vi "Run Alicat Configuration.vi"(8 "error in (no error)":errorcluster, 11 "Alicat Device in":refnum<class "Alicat Device.lvclass">) -> (0 "error out":errorcluster, 1 "value":dbl, 2 "Accessors:controller_":bool, 3 "Alicat Device out":refnum<class "Alicat Device.lvclass">)   [LabVIEW 2014, in "Alicat Lib.lvlib" / "Alicat Device.lvclass"]
uses:
  Alicat Device.lvclass
  reusable/Session APIs/Serial/Serial Session.lvclass
  Data/Alicat Data.lvclass
  Configurable Device/Configurable Device.lvclass/Configurable Device.ctl
  reusable/Data/Data.lvclass/Data.ctl
  Data/Alicat Data.lvclass/Alicat Data.ctl
  Alicat Device.lvclass/Alicat Device.ctl
  reusable/Session APIs/File Access/Config Data/Config Data.lvclass/Config Data.ctl
  Configurable Device/Accessors/Write label.vi
  Accessors/Read Session Handle.vi
  Configurable Device/Read controller_.vi
  Accessors/Write Session Handle.vi
  Configurable Device/Accessors/Write type.vi
  reusable/Data/Write Data ID.vi
  Data/Accessors/Write ID.vi
  Configurable Device/Read Handle.vi
  Configurable Device/Read Log Session.vi
  <vilib>/Utility/config.llb/Read Key (String).vi
  <vilib>/Utility/config.llb/Read Key (Double).vi
  reusable/Session APIs/File Access/Config Data/Config Data.lvclass
  <userlib>/_Session Fwk/Session - Root.lvclass
  <vilib>/ErrorRing/Error Ring.xnode
  <vilib>/Utility/config.llb/NI_LVConfig.lvlib
  Configurable Device/Configurable Device.lvclass
  reusable/Session APIs/Session Log/System Log.lvclass
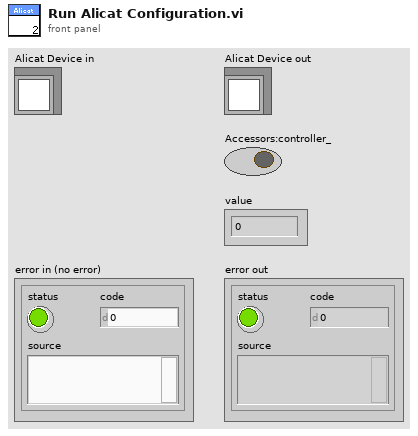
[diagram p1: front panel]
types:
  T1 = typedef "Serial Session.lvclass/Session Handle.ctl" = refnum<data-value>
  T2 = typedef "Config Data.lvclass/Config Session.ctl" = refnum<data-value>
  T3 = typedef "Session - Root.lvclass/Session Handle.ctl" = refnum<data-value>
  T4 = typedef "NI_LVConfig.lvlib/Config Data RefNum.ctl" = refnum<k1>
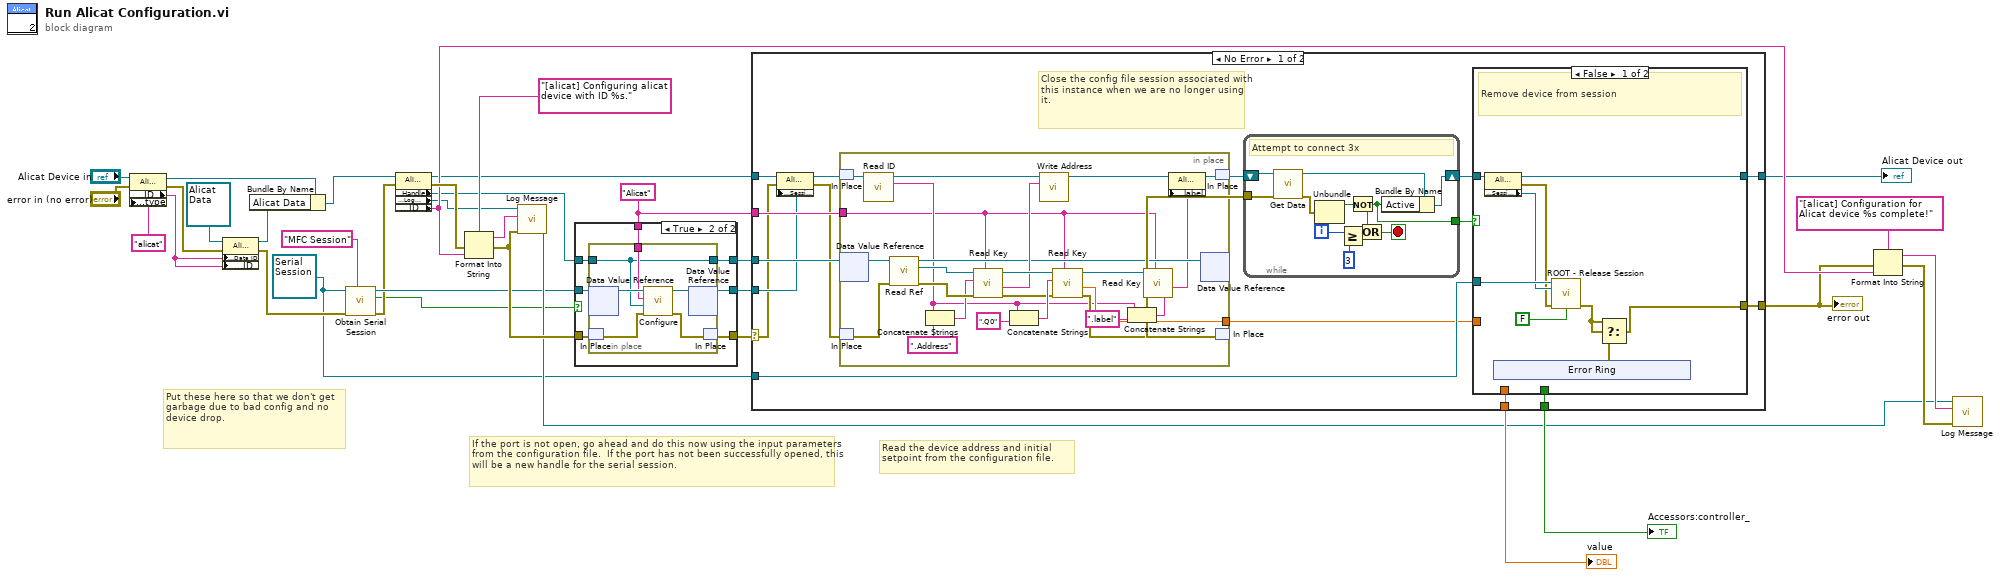
[diagram p0: block diagram]
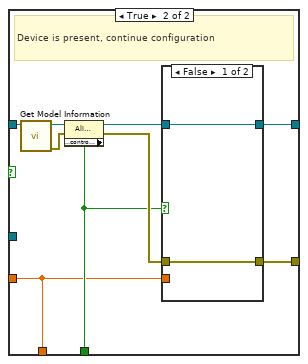
[diagram p2: hidden frame]
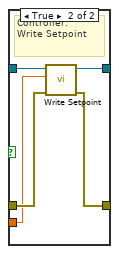
[diagram p3: hidden frame]
diagram:
  w8 = refnum<class "Serial Session.lvclass"> refnum ("Serial Session in")
  w6 = "Alicat" ("section")
  # "Put these here so that we don't get garbage due to bad config and no device drop."
  # "If the port is not open, go ahead and do this now using the input parameters from the configuration file.  If the port has not been successfully opened, this will be a new handle for the serial session."
  # "Read the device address and initial setpoint from the configuration file."
  n1 = property class="Alicat Device"(reference="Alicat Device in", error in="error in (no error)", "Accessors:type"="alicat" ("type")) -> (reference out=w24:refnum<class "Alicat Device.lvclass">, error out=w27:errorcluster, "Accessors:ID"=w23:string)
  n2 = property class="Alicat Data"(reference=refnum<class "Alicat Data.lvclass"> refnum ("Alicat Lib.lvlib:Alicat Data"), error in=w27, "Accessors:Data ID"=w23, "Accessors:ID"=w23) -> (reference out=w26:refnum<class "Alicat Data.lvclass">, error out=w28:errorcluster)
  n3 = Bundle By Name(cluster=w24, "Alicat Data"=w26) -> (w25:refnum<class "Alicat Device.lvclass">)
  n4 = call "Obtain Serial Session.vi"("Session Name ()"="MFC Session", "error in"=w28, "Serial Session in"=w8) -> ("error out"=w4:errorcluster, "created new?"=w1:bool, "hSerial"=w7:T1)  [unwired: 6 in]
  n5 = property class="Alicat Device"(reference=w25, error in=w4) -> (reference out=w9:refnum<class "Alicat Device.lvclass">, error out=w29:errorcluster, "Accessors:Handle"=w3:T2, "Accessors:Log Session"=w13:T3, "Accessors:ID"=w21:string)
  n6 = Format Into String(format string="[alicat] Configuring alicat device with ID %s.", error in=w29, w21) -> (resulting string=w15:string, error out=w30:errorcluster)  [unwired: 1 in]
  n7 = call "Log Message.vi"("error in"=w30, "MSG In"=w15, "session in"=w13) -> ("session out"=w16:T3)  [unwired: 7 in, 1 out]
  n8 = case shown="True" w1 {
    tunnel: w7 -> [w38 w45]
    tunnel: w30 -> [w37 w41]
    tunnel: [w38 w44] -> w10
    tunnel: [w37 w43] -> w11
    tunnel: w3 -> [w36 w42]
    tunnel: [w36 w40] -> w5
    tunnel: w6 -> [_ w39]
    frame False {
    }
    frame True {
      n9 = in-place {
        in-place-border: w42 -> [w46]
        in-place-border: w39 -> [w47]
        in-place-border: [w46] -> w40
        n10 = in-place-dvr #1(w45) -> (w51:refnum<class "Serial Session.lvclass">)  [unwired: 1 out]
        n11 = in-place-match #2(w41) -> (w50:errorcluster)
        n12 = call "Configure.vi"("error in"=w50, "Config Handle"=w46, "section"=w47, "Serial Session in"=w51) -> ("error out"=w49:errorcluster, "Serial Session out"=w48:refnum<class "Serial Session.lvclass">)  [unwired: 6 in]
        n13 = in-place-dvr #1(w48) -> (w44:T1)  [unwired: 1 out]
        n14 = in-place-match #2(w49) -> (w43:errorcluster)
      }
    }
  }
  n15 = case shown="No Error" w11 {
    selector: w11 -> [w56 w130]
    tunnel: w5 -> [w68 _]
    tunnel: w6 -> [w67 _]
    tunnel: w8 -> [w66 _]
    tunnel: [w64 w130] -> w20
    tunnel: [w61 w131] -> w12
    tunnel: w9 -> [w60 w131]
    tunnel: w10 -> [w58 _]
    tunnel: [w53 _] -> w34
    tunnel: [w52 _] -> w35
    frame No Error {
      # "Close the config file session associated with this instance when we are no longer using it."
      n16 = property class="Alicat Device"(reference=w60, error in=w56, "Accessors:Session Handle"=w58) -> (reference out=w59:refnum<class "Alicat Device.lvclass">, error out=w57:errorcluster)
      n17 = in-place {
        in-place-border: w67 -> [w106]
        in-place-border: [w118] -> w62
        n18 = in-place-match #3(w59) -> (w116:refnum<class "Alicat Device.lvclass">)
        n19 = in-place-dvr #4(w68) -> (w129:refnum<class "Config Data.lvclass">)  [unwired: 1 out]
        n20 = in-place-match #5(w57) -> (w128:errorcluster)
        n21 = call "Read ID.vi"("Configurable Device in"=w116) -> ("ID"=w109:string, "Configurable Device out"=w115:refnum<class "Alicat Device.lvclass">)  [unwired: 8 in, 1 out]
        n22 = call "Read Ref.vi"("error in"=w128, "Config Data in"=w129) -> ("error out"=w126:errorcluster, "config data"=w127:T4, "Config Data out"=w117:refnum<class "Config Data.lvclass">)  [unwired: 7 in]
        n23 = Concatenate Strings(w109, ".Address" ("string")) -> (w124:string)
        n24 = call-poly <vilib>:"Read Key.vi"("section"=w106, "error in (no error)"=w126, "key"=w124, "refnum"=w127) -> ("error out"=w120:errorcluster, "value"=w119:string, "refnum out"=w123:T4)  [unwired: 4 in, 1 out]
        n25 = Concatenate Strings(w109, ".Q0" ("string")) -> (w121:string)
        n26 = call "Write Address.vi"("Address"=w119, "Alicat Device in"=w115) -> ("Alicat Device out"=w113:refnum<class "Alicat Device.lvclass">)  [unwired: 8 in, 1 out]
        n27 = call-poly <vilib>:"Read Key.vi"("section"=w106, "error in (no error)"=w120, "key"=w121, "refnum"=w123) -> ("error out"=w114:errorcluster, "value"=w118:dbl, "refnum out"=w108:T4)  [unwired: 4 in, 1 out]
        n28 = Concatenate Strings(w109, ".label" ("string")) -> (w110:string)
        n29 = call-poly <vilib>:"Read Key.vi"("section"=w106, "key"=w110, "refnum"=w108) -> ("value"=w107:string)  [unwired: 5 in, 3 out]
        n30 = property class="Alicat Device"(reference=w113, "Accessors:label"=w107) -> (reference out=w112:refnum<class "Alicat Device.lvclass">)  [unwired: 1 in, 1 out]
        n31 = in-place-dvr #4(w117) -> ()  [unwired: 2 out]
        n32 = in-place-match #3(w112) -> (w65:refnum<class "Alicat Device.lvclass">)
        n33 = in-place-match #5(w114) -> (w54:errorcluster)
      }
      n34 = while {
        tunnel: w54 -> [w100]
        shift-right: [w98] -> w63
        shift-left: w65 -> [w101]
        tunnel: [w97] -> w55
        i -> [w95]
        stop <- w102 stop-if-true
        # "Attempt to connect 3x"
        n35 = call-dynamic "Get Data.vi"("error in"=w100, "Alicat Device in"=w101) -> ("error out"=w96:errorcluster, "Alicat Device out"=w99:refnum<class "Alicat Device.lvclass">)  [unwired: 7 in, 1 out]
        n36 = Unbundle(w96) -> ("status"=w103:bool)  [unwired: 2 out]
        n37 = Greater Or Equal?(x=w95, y=3) -> (x >= y?=w104:bool)
        n38 = Not(x=w103) -> (.not. x?=w97:bool)
        n39 = Or(x=w97, y=w104) -> (x .or. y?=w102:bool)
        n40 = Bundle By Name(cluster=w99, "Active"=w97) -> (w98:refnum<class "Alicat Device.lvclass">)
      }
      n41 = case shown="False" w55 {
        tunnel: [w69 w86] -> w64
        tunnel: w66 -> [w77 _]
        tunnel: w63 -> [w75 w87]
        tunnel: w62 -> [_ w79]
        tunnel: [w74 w85] -> w61
        tunnel: [_ w80] -> w53
        tunnel: [_ w79] -> w52
        frame False {
          # "Remove device from session"
          n42 = property class="Alicat Device"(reference=w75) -> (reference out=w74:refnum<class "Alicat Device.lvclass">, error out=w72:errorcluster, "Accessors:Session Handle"=w73:T1)  [unwired: 1 in]
          n43 = xnode "Error Ring"() -> ("error out"=w70:errorcluster)
          n44 = call <userlib>:"ROOT - Release Session.vi"("OBJ - Session in"=w77, "Session Handle in"=w73, "error in (no error)"=w72, "force destroy? (F)"=FALSE) -> ("error out"=w71:errorcluster)  [unwired: 10 in, 1 out]
          n45 = Select(t=w71, s=w71, f=w70) -> (s? t:f=w69:errorcluster)
        }
        frame True {
          # "Device is present, continue configuration"
          n46 = call "Get Model Information.vi"("Alicat Device in"=w87) -> ("error out"=w81:errorcluster, "Alicat Device out"=w84:refnum<class "Alicat Device.lvclass">)  [unwired: 7 in, 2 out]
          n47 = property class="Alicat Device"(reference=w84, error in=w81) -> (reference out=w83:refnum<class "Alicat Device.lvclass">, error out=w82:errorcluster, "Accessors:controller_"=w80:bool)
          n48 = case shown="False" w80 {
            tunnel: w82 -> [w88 w93]
            tunnel: w83 -> [w89 w94]
            tunnel: w79 -> [_ w90]
            tunnel: [w88 w92] -> w86
            tunnel: [w89 w91] -> w85
            frame False {
            }
            frame True {
              # "Controller:\nWrite Setpoint"
              n49 = call "Write Setpoint.vi"("error in"=w93, "Setpoint"=w90, "Alicat Device in"=w94) -> ("error out"=w92:errorcluster, "Alicat Device out"=w91:refnum<class "Alicat Device.lvclass">)  [unwired: 6 in, 1 out]
            }
          }
        }
      }
    }
    frame Error {
    }
  }
  "value" <- w35
  "Accessors:controller_" <- w34
  "error out" <- w20
  "Alicat Device out" <- w12
  n50 = Format Into String(format string="[alicat] Configuration for Alicat device %s complete!", error in=w20, w21) -> (resulting string=w18:string, error out=w19:errorcluster)  [unwired: 1 in]
  n51 = call "Log Message.vi"("error in"=w19, "MSG In"=w18, "session in"=w16) -> ()  [unwired: 7 in, 2 out]
